vi "History.vi"(8 "error in":errorcluster, 9 "time":u32, 10 "Value":dbl, 11 "variant in":variant) -> (0 "error out":errorcluster, 3 "variant out":variant, 4 "history graph":cluster{dbl[], dbl[]})   [LabVIEW 2013]
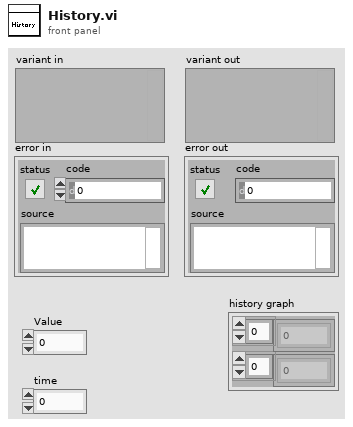
[diagram p1: front panel]
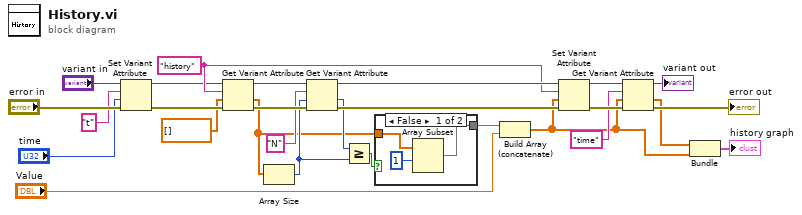
[diagram p0: block diagram]
diagram:
  w14 = "history" ("name")
  n1 = Set Variant Attribute(Variant="variant in", name="t", value="time", error in="error in") -> (Variant out=w9:variant, error out=w22:errorcluster)  [unwired: 1 out]
  n2 = Get Variant Attribute(Variant=w9, name=w14, default value (empty Variant)=dbl[] [], error in=w22) -> (duplicate Variant=w15:variant, value=w12:dbl[], error out=w23:errorcluster)  [unwired: 1 out]
  n3 = Array Size(array=w12) -> (size(s)=w18:i32)
  n4 = Get Variant Attribute(Variant=w15, name="N", default value (empty Variant)=w18, error in=w23) -> (duplicate Variant=w16:variant, value=w19:i32, error out=w24:errorcluster)  [unwired: 1 out]
  n5 = Greater Or Equal?(x=w19, y=w18) -> (x >= y?=w11:bool)
  n6 = case shown="False" w11 {
    tunnel: w12 -> [w30 w31]
    tunnel: [w29 w31] -> w13
    frame False {
      n7 = Array Subset(array=w30, index=1) -> (w29:dbl[])  [unwired: 1 in]
    }
    frame True {
    }
  }
  n8 = Build Array (concatenate)(w13, "Value") -> (w4:dbl[])
  n9 = Set Variant Attribute(Variant=w16, name=w14, value=w4, error in=w24) -> (Variant out=w20:variant, error out=w25:errorcluster)  [unwired: 1 out]
  n10 = Get Variant Attribute(Variant=w20, name="time", default value (empty Variant)=w4, error in=w25) -> (duplicate Variant=→"variant out":variant, value=w5:dbl[], error out=→"error out":errorcluster)  [unwired: 1 out]
  n11 = Bundle(w5, w4) -> (→"history graph":cluster{dbl[], dbl[]})  [unwired: 1 in]
